vi "GetHighPrioritySensors.vi"() -> ()   [LabVIEW 2019]
uses:
  refnums.vi
  sensors.vi
  dsdata.vi
  <vilib>/Utility/xml.llb/Write to XML File(string).vi
  <vilib>/Utility/xml.llb/Read From XML File(array).vi
panel:
  in  "Plot":bool
  out "Drive Encoder Velocities":T1(graph)
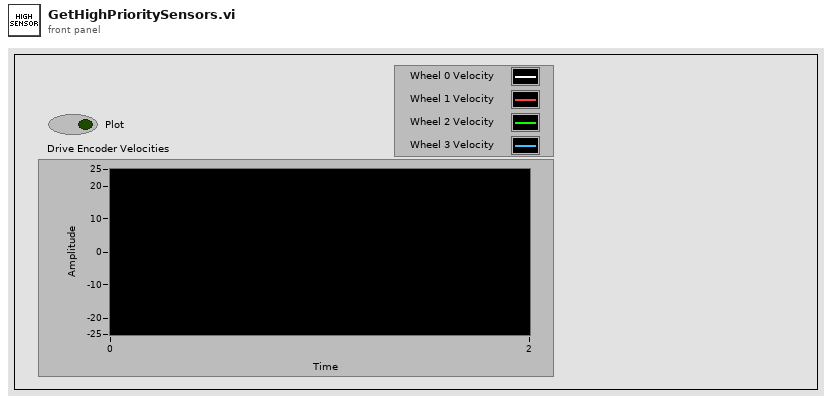
[diagram p1: front panel]
types:
  T1 = cluster{"Sensor Velocity":dbl, "Sensor Velocity":dbl, "Sensor Velocity":dbl, "Sensor Velocity":dbl}
  T2 = typedef "WPI_MotorControlDeviceRef.ctl" = cluster{"DeviceStatus":errorcluster, "Type":T3, "PWM":cluster{"PWM Channel":T4, "DeadBand":T5}, "CAN":cluster{"Device Number":u8, "SetOutput VI Ref":variant, "GetOutput VI Ref":variant, "Enable VI Ref":variant, "Disable VI Ref":variant, "Data":variant}, "Invert":bool, "DIO PWM":cluster{"PWM \"Enable\" Channel":T4, "DIOChannel":T6, "PWM Rate":dbl}}
  T3 = typedef "WPI_MotorControlType.ctl" = enum16{"PWM", "CAN", "DIO PWM"}
  T4 = typedef "FPGA_DIOPWMChannel.ctl" = enum8{"PWM 0", "PWM 1", "PWM 2", "PWM 3", "PWM 4", "PWM 5", "PWM 6", "PWM 7", "PWM 8", "PWM 9", "PWM MXP 0", "PWM MXP 1", "PWM MXP 2", "PWM MXP 3", "PWM MXP 4", "PWM MXP 5", "PWM MXP 6", "PWM MXP 7", "PWM MXP 8", "PWM MXP 9", "Invalid"}
  T5 = typedef "WPI_PWMDeadband.ctl" = cluster{"Name":string, "maxPositivePwm":i32, "minPositivePwm":i32, "centerPwm":i32, "maxNegativePwm":i32, "minNegativePwm":i32, "angularRange":u16}
  T6 = typedef "FPGA_DIOChannel.ctl" = enum8{"DIO 0", "DIO 1", "DIO 2", "DIO 3", "DIO 4", "DIO 5", "DIO 6", "DIO 7", "DIO 8", "DIO 9", "DIO MXP 0", "DIO MXP 1", "DIO MXP 2", "DIO MXP 3", "DIO MXP 4", "DIO MXP 5", "DIO MXP 6", "DIO MXP 7", "DIO MXP 8", "DIO MXP 9", "DIO MXP 10", "DIO MXP 11", "DIO MXP 12", "DIO MXP 13", "DIO MXP 14", "DIO MXP 15", "SPI Port CS1", "SPI Port CS2", "SPI Port CS3", "SPI Port MISO", "SPI Port MOSI", "Invalid"}
  T7 = typedef "WPI_PotentiometerDevRef.ctl" = cluster{"DevStatus":errorcluster, "Analog Channel":T8, "Invert Output":bool}
  T8 = typedef "FPGA_AIChannel.ctl" = enum8{"AI 0", "AI 1", "AI 2", "AI 3", "AI MXP 0", "AI MXP 1", "AI MXP 2", "AI MXP 3", "Invalid"}
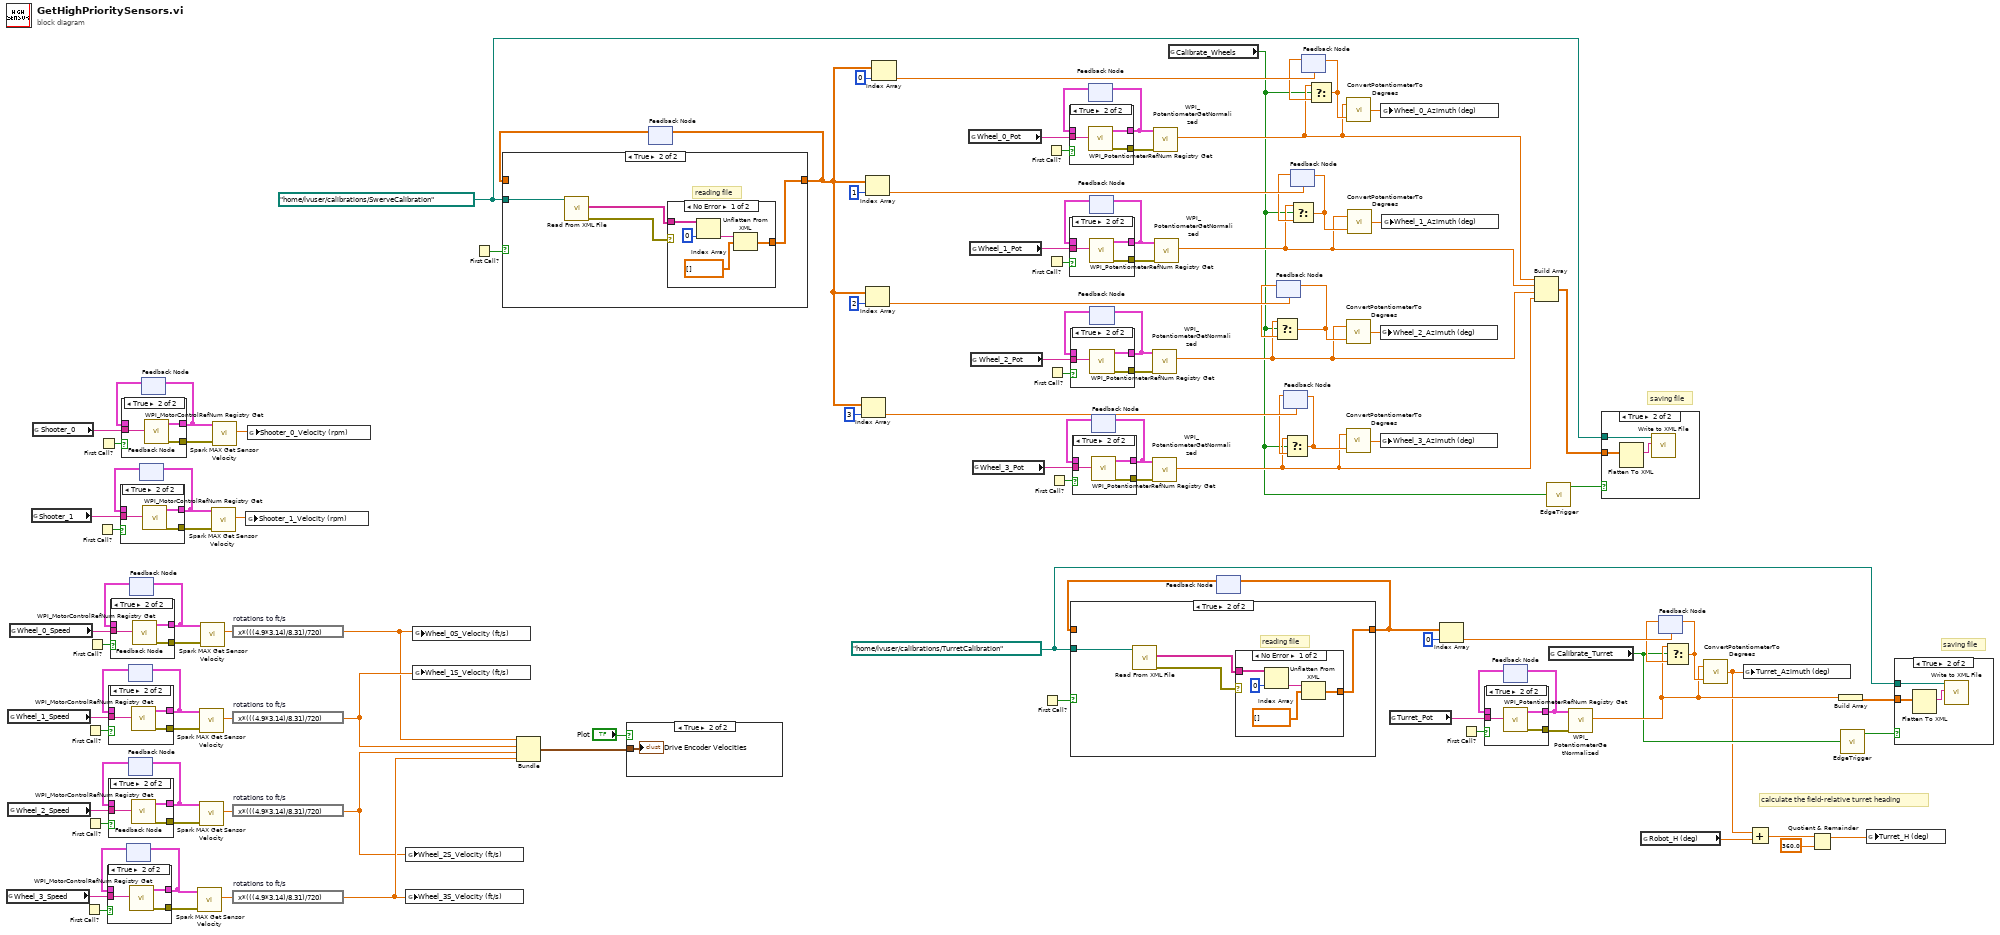
[diagram p0: block diagram]
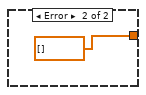
[diagram p4: hidden frame]
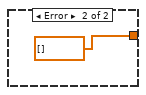
[diagram p15: hidden frame]
diagram:
  w8 = path "/home/lvuser/calibrations/TurretCalibration" ("path")
  w67 = path "/home/lvuser/calibrations/SwerveCalibration" ("path")
  # "calculate the field-relative turret heading"
  # "saving file"
  # "saving file"
  n1 = global read "refnums.vi" "Wheel_3_Speed"() -> (w33:string)
  n2 = global read "refnums.vi" "Wheel_1_Speed"() -> (w43:string)
  n3 = global read "refnums.vi" "Wheel_2_Speed"() -> (w38:string)
  n4 = global read "refnums.vi" "Wheel_0_Speed"() -> (w48:string)
  n5 = global read "refnums.vi" "Shooter_1"() -> (w56:string)
  n6 = global read "refnums.vi" "Shooter_0"() -> (w62:string)
  n7 = First Call?() -> (First Call?: T/F=w35:bool)
  n8 = First Call?() -> (First Call?: T/F=w45:bool)
  n9 = First Call?() -> (First Call?: T/F=w40:bool)
  n10 = First Call?() -> (First Call?: T/F=w50:bool)
  n11 = First Call?() -> (First Call?: T/F=w58:bool)
  n12 = First Call?() -> (First Call?: T/F=w64:bool)
  n13 = feedback #1() -> (w34:T2)  [unwired: 1 in]
  n14 = case shown="True" w35 {
    tunnel: [w116 w119] -> w31
    tunnel: w34 -> [w116 _]
    tunnel: w33 -> [_ w117]
    tunnel: [_ w118] -> w32
    frame False {
    }
    frame True {
      n15 = call <vilib>:"WPI_MotorControlRefNum Registry Get.vi"("refnum name"=w117) -> ("error out"=w118:errorcluster, "MotorControlDevRef"=w119:T2)  [unwired: 9 in]
    }
  }
  n16 = feedback-in #1(w31) -> ()
  n17 = feedback #2() -> (w44:T2)  [unwired: 1 in]
  n18 = case shown="True" w45 {
    tunnel: [w120 w123] -> w41
    tunnel: w44 -> [w120 _]
    tunnel: w43 -> [_ w121]
    tunnel: [_ w122] -> w42
    frame False {
    }
    frame True {
      n19 = call <vilib>:"WPI_MotorControlRefNum Registry Get.vi"("refnum name"=w121) -> ("error out"=w122:errorcluster, "MotorControlDevRef"=w123:T2)  [unwired: 9 in]
    }
  }
  n20 = feedback-in #2(w41) -> ()
  n21 = feedback #3() -> (w39:T2)  [unwired: 1 in]
  n22 = case shown="True" w40 {
    tunnel: [w124 w127] -> w36
    tunnel: w39 -> [w124 _]
    tunnel: w38 -> [_ w125]
    tunnel: [_ w126] -> w37
    frame False {
    }
    frame True {
      n23 = call <vilib>:"WPI_MotorControlRefNum Registry Get.vi"("refnum name"=w125) -> ("error out"=w126:errorcluster, "MotorControlDevRef"=w127:T2)  [unwired: 9 in]
    }
  }
  n24 = feedback-in #3(w36) -> ()
  n25 = feedback #4() -> (w49:T2)  [unwired: 1 in]
  n26 = case shown="True" w50 {
    tunnel: [w128 w131] -> w46
    tunnel: w49 -> [w128 _]
    tunnel: w48 -> [_ w129]
    tunnel: [_ w130] -> w47
    frame False {
    }
    frame True {
      n27 = call <vilib>:"WPI_MotorControlRefNum Registry Get.vi"("refnum name"=w129) -> ("error out"=w130:errorcluster, "MotorControlDevRef"=w131:T2)  [unwired: 9 in]
    }
  }
  n28 = feedback-in #4(w46) -> ()
  n29 = feedback #5() -> (w57:T2)  [unwired: 1 in]
  n30 = case shown="True" w58 {
    tunnel: [w132 w135] -> w54
    tunnel: w57 -> [w132 _]
    tunnel: w56 -> [_ w133]
    tunnel: [_ w134] -> w55
    frame False {
    }
    frame True {
      n31 = call <vilib>:"WPI_MotorControlRefNum Registry Get.vi"("refnum name"=w133) -> ("error out"=w134:errorcluster, "MotorControlDevRef"=w135:T2)  [unwired: 9 in]
    }
  }
  n32 = feedback-in #5(w54) -> ()
  n33 = feedback #6() -> (w63:T2)  [unwired: 1 in]
  n34 = case shown="True" w64 {
    tunnel: [w136 w139] -> w60
    tunnel: w63 -> [w136 _]
    tunnel: w62 -> [_ w137]
    tunnel: [_ w138] -> w61
    frame False {
    }
    frame True {
      n35 = call <vilib>:"WPI_MotorControlRefNum Registry Get.vi"("refnum name"=w137) -> ("error out"=w138:errorcluster, "MotorControlDevRef"=w139:T2)  [unwired: 9 in]
    }
  }
  n36 = feedback-in #6(w60) -> ()
  n37 = call <vilib>:"Spark MAX Get Sensor Velocity.vi"("error in (no error)"=w32, "MotorControlDevRef in"=w31) -> ("Sensor Velocity"=w30:dbl)  [unwired: 6 in, 3 out]
  n38 = call <vilib>:"Spark MAX Get Sensor Velocity.vi"("error in (no error)"=w42, "MotorControlDevRef in"=w41) -> ("Sensor Velocity"=w26:dbl)  [unwired: 6 in, 3 out]
  n39 = call <vilib>:"Spark MAX Get Sensor Velocity.vi"("error in (no error)"=w37, "MotorControlDevRef in"=w36) -> ("Sensor Velocity"=w28:dbl)  [unwired: 6 in, 3 out]
  n40 = call <vilib>:"Spark MAX Get Sensor Velocity.vi"("error in (no error)"=w47, "MotorControlDevRef in"=w46) -> ("Sensor Velocity"=w23:dbl)  [unwired: 6 in, 3 out]
  n41 = call <vilib>:"Spark MAX Get Sensor Velocity.vi"("error in (no error)"=w55, "MotorControlDevRef in"=w54) -> ("Sensor Velocity"=w53:dbl)  [unwired: 6 in, 3 out]
  n42 = call <vilib>:"Spark MAX Get Sensor Velocity.vi"("error in (no error)"=w61, "MotorControlDevRef in"=w60) -> ("Sensor Velocity"=w59:dbl)  [unwired: 6 in, 3 out]
  n43 = expression code="x*(((4.9*3.14)/8.31)/720)" "rotations to ft/s"(w23) -> (w24:dbl)
  n44 = expression code="x*(((4.9*3.14)/8.31)/720)" "rotations to ft/s"(w26) -> (w25:dbl)
  n45 = expression code="x*(((4.9*3.14)/8.31)/720)" "rotations to ft/s"(w28) -> (w27:dbl)
  n46 = expression code="x*(((4.9*3.14)/8.31)/720)" "rotations to ft/s"(w30) -> (w29:dbl)
  n47 = global write "sensors.vi" "Shooter_1_Velocity (rpm)"(w53) -> ()
  n48 = global write "sensors.vi" "Shooter_0_Velocity (rpm)"(w59) -> ()
  n49 = global write "sensors.vi" "Wheel_2S_Velocity (ft/s)"(w27) -> ()
  n50 = global write "sensors.vi" "Wheel_3S_Velocity (ft/s)"(w29) -> ()
  n51 = global write "sensors.vi" "Wheel_0S_Velocity (ft/s)"(w24) -> ()
  n52 = global write "sensors.vi" "Wheel_1S_Velocity (ft/s)"(w25) -> ()
  n53 = First Call?() -> (First Call?: T/F=w73:bool)
  n54 = Bundle("Sensor Velocity"=w24, "Sensor Velocity"=w25, "Sensor Velocity"=w27, "Sensor Velocity"=w29) -> (w52:T1)  [unwired: 1 in]
  n55 = case shown="True" "Plot" {
    tunnel: w52 -> [_ w140]
    frame False {
    }
    frame True {
      "Drive Encoder Velocities" <- w140
    }
  }
  n56 = feedback #7() -> (w88:dbl[])  [unwired: 1 in]
  n57 = case shown="True" w73 {
    tunnel: w67 -> [_ w145]
    tunnel: [w141 w142] -> w79
    tunnel: w88 -> [w141 _]
    frame False {
    }
    frame True {
      # "reading file"
      n58 = call-poly <vilib>:"Read From XML File.vi"("XML File Path"=w145) -> ("error out"=w143:errorcluster, "XML Elements"=w144:string[])  [unwired: 8 in, 1 out]
      n59 = case shown="No Error" w143 {
        tunnel: w144 -> [w149 _]
        tunnel: [w147 dbl[] [] ("appended array")] -> w142
        frame No Error {
          n60 = Index Array(array=w149, index=0) -> (element=w148:string)
          n61 = Unflatten From XML(xml string=w148, type=dbl[] [] ("appended array")) -> (value=w147:dbl[])  [unwired: 1 in, 1 out]
        }
        frame Error {
        }
      }
    }
  }
  n62 = feedback-in #7(w79) -> ()
  n63 = Index Array(array=w79, index=3) -> (element=w81:dbl)
  n64 = Index Array(array=w79, index=1) -> (element=w86:dbl)
  n65 = Index Array(array=w79, index=2) -> (element=w83:dbl)
  n66 = Index Array(array=w79, index=0) -> (element=w90:dbl)
  n67 = global read "refnums.vi" "Wheel_0_Pot"() -> (w109:string)
  n68 = global read "refnums.vi" "Wheel_1_Pot"() -> (w105:string)
  n69 = global read "refnums.vi" "Wheel_2_Pot"() -> (w99:string)
  n70 = global read "refnums.vi" "Wheel_3_Pot"() -> (w94:string)
  n71 = First Call?() -> (First Call?: T/F=w11:bool)
  n72 = First Call?() -> (First Call?: T/F=w111:bool)
  n73 = First Call?() -> (First Call?: T/F=w107:bool)
  n74 = First Call?() -> (First Call?: T/F=w101:bool)
  n75 = First Call?() -> (First Call?: T/F=w96:bool)
  n76 = feedback #8() -> (w110:T7)  [unwired: 1 in]
  n77 = case shown="True" w111 {
    tunnel: [w152 w154] -> w108
    tunnel: w110 -> [w152 _]
    tunnel: w109 -> [_ w155]
    tunnel: [_ w153] -> w104
    frame False {
    }
    frame True {
      n78 = call <vilib>:"WPI_PotentiometerRefNum Registry Get.vi"("refnum name"=w155) -> ("error out"=w153:errorcluster, "PotDevRef"=w154:T7)  [unwired: 9 in]
    }
  }
  n79 = feedback-in #8(w108) -> ()
  n80 = feedback #9() -> (w106:T7)  [unwired: 1 in]
  n81 = case shown="True" w107 {
    tunnel: [w156 w158] -> w103
    tunnel: w106 -> [w156 _]
    tunnel: w105 -> [_ w159]
    tunnel: [_ w157] -> w102
    frame False {
    }
    frame True {
      n82 = call <vilib>:"WPI_PotentiometerRefNum Registry Get.vi"("refnum name"=w159) -> ("error out"=w157:errorcluster, "PotDevRef"=w158:T7)  [unwired: 9 in]
    }
  }
  n83 = feedback-in #9(w103) -> ()
  n84 = feedback #10() -> (w100:T7)  [unwired: 1 in]
  n85 = case shown="True" w101 {
    tunnel: [w160 w162] -> w98
    tunnel: w100 -> [w160 _]
    tunnel: w99 -> [_ w163]
    tunnel: [_ w161] -> w97
    frame False {
    }
    frame True {
      n86 = call <vilib>:"WPI_PotentiometerRefNum Registry Get.vi"("refnum name"=w163) -> ("error out"=w161:errorcluster, "PotDevRef"=w162:T7)  [unwired: 9 in]
    }
  }
  n87 = feedback-in #10(w98) -> ()
  n88 = feedback #11() -> (w95:T7)  [unwired: 1 in]
  n89 = case shown="True" w96 {
    tunnel: [w164 w166] -> w93
    tunnel: w95 -> [w164 _]
    tunnel: w94 -> [_ w167]
    tunnel: [_ w165] -> w92
    frame False {
    }
    frame True {
      n90 = call <vilib>:"WPI_PotentiometerRefNum Registry Get.vi"("refnum name"=w167) -> ("error out"=w165:errorcluster, "PotDevRef"=w166:T7)  [unwired: 9 in]
    }
  }
  n91 = feedback-in #11(w93) -> ()
  n92 = call <vilib>:"WPI_PotentiometerGetNormalized.vi"("error in"=w97, "PotDevRef"=w98) -> ("Normalized Value"=w70:dbl)  [unwired: 7 in, 2 out]
  n93 = call <vilib>:"WPI_PotentiometerGetNormalized.vi"("error in"=w92, "PotDevRef"=w93) -> ("Normalized Value"=w69:dbl)  [unwired: 7 in, 2 out]
  n94 = call <vilib>:"WPI_PotentiometerGetNormalized.vi"("error in"=w104, "PotDevRef"=w108) -> ("Normalized Value"=w68:dbl)  [unwired: 7 in, 2 out]
  n95 = call <vilib>:"WPI_PotentiometerGetNormalized.vi"("error in"=w102, "PotDevRef"=w103) -> ("Normalized Value"=w71:dbl)  [unwired: 7 in, 2 out]
  n96 = global read "dsdata.vi" "Calibrate_Wheels"() -> (w66:bool)
  n97 = feedback #12() -> (w14:dbl[])  [unwired: 1 in]
  n98 = case shown="True" w11 {
    tunnel: w8 -> [_ w172]
    tunnel: [w168 w169] -> w13
    tunnel: w14 -> [w168 _]
    frame False {
    }
    frame True {
      # "reading file"
      n99 = call-poly <vilib>:"Read From XML File.vi"("XML File Path"=w172) -> ("error out"=w170:errorcluster, "XML Elements"=w171:string[])  [unwired: 8 in, 1 out]
      n100 = case shown="No Error" w170 {
        tunnel: w171 -> [w176 _]
        tunnel: [w174 dbl[] [] ("appended array")] -> w169
        frame No Error {
          n101 = Index Array(array=w176, index=0) -> (element=w175:string)
          n102 = Unflatten From XML(xml string=w175, type=dbl[] [] ("appended array")) -> (value=w174:dbl[])  [unwired: 1 in, 1 out]
        }
        frame Error {
        }
      }
    }
  }
  n103 = feedback-in #12(w13) -> ()
  n104 = feedback #13(w83) -> (w82:dbl)
  n105 = Select(t=w70, s=w66, f=w82) -> (s? t:f=w75:dbl)
  n106 = feedback-in #13(w75) -> ()
  n107 = feedback #14(w81) -> (w80:dbl)
  n108 = Select(t=w69, s=w66, f=w80) -> (s? t:f=w74:dbl)
  n109 = feedback-in #14(w74) -> ()
  n110 = feedback #15(w86) -> (w85:dbl)
  n111 = Select(t=w71, s=w66, f=w85) -> (s? t:f=w76:dbl)
  n112 = feedback-in #15(w76) -> ()
  n113 = feedback #16(w90) -> (w89:dbl)
  n114 = Select(t=w68, s=w66, f=w89) -> (s? t:f=w77:dbl)
  n115 = feedback-in #16(w77) -> ()
  n116 = call "ConvertPotentiometerToDegrees.vi"("Forward Position Wheel 1 [0-1]"=w75, "Raw Potentiometer Value"=w70) -> ("Orientation (deg)"=w113:dbl)
  n117 = call "ConvertPotentiometerToDegrees.vi"("Forward Position Wheel 1 [0-1]"=w74, "Raw Potentiometer Value"=w69) -> ("Orientation (deg)"=w112:dbl)
  n118 = call "ConvertPotentiometerToDegrees.vi"("Forward Position Wheel 1 [0-1]"=w77, "Raw Potentiometer Value"=w68) -> ("Orientation (deg)"=w115:dbl)
  n119 = call "ConvertPotentiometerToDegrees.vi"("Forward Position Wheel 1 [0-1]"=w76, "Raw Potentiometer Value"=w71) -> ("Orientation (deg)"=w114:dbl)
  n120 = global write "sensors.vi" "Wheel_2_Azimuth (deg)"(w113) -> ()
  n121 = global write "sensors.vi" "Wheel_3_Azimuth (deg)"(w112) -> ()
  n122 = global write "sensors.vi" "Wheel_0_Azimuth (deg)"(w115) -> ()
  n123 = global write "sensors.vi" "Wheel_1_Azimuth (deg)"(w114) -> ()
  n124 = global read "refnums.vi" "Turret_Pot"() -> (w20:string)
  n125 = Index Array(array=w13, index=0) -> (element=w16:dbl)
  n126 = First Call?() -> (First Call?: T/F=w22:bool)
  n127 = feedback #17() -> (w21:T7)  [unwired: 1 in]
  n128 = case shown="True" w22 {
    tunnel: [w179 w181] -> w19
    tunnel: w21 -> [w179 _]
    tunnel: w20 -> [_ w182]
    tunnel: [_ w180] -> w18
    frame False {
    }
    frame True {
      n129 = call <vilib>:"WPI_PotentiometerRefNum Registry Get.vi"("refnum name"=w182) -> ("error out"=w180:errorcluster, "PotDevRef"=w181:T7)  [unwired: 9 in]
    }
  }
  n130 = feedback-in #17(w19) -> ()
  n131 = Build Array(w68, w71, w70, w69) -> (w72:dbl[])
  n132 = call "EdgeTrigger.vi"("Input Signal"=w66) -> ("Rising Edge Trigger"=w65:bool)  [unwired: 2 out]
  n133 = global read "dsdata.vi" "Calibrate_Turret"() -> (w6:bool)
  n134 = call <vilib>:"WPI_PotentiometerGetNormalized.vi"("error in"=w18, "PotDevRef"=w19) -> ("Normalized Value"=w9:dbl)  [unwired: 7 in, 2 out]
  n135 = case shown="True" w65 {
    tunnel: w67 -> [_ w185]
    tunnel: w72 -> [_ w184]
    frame False {
    }
    frame True {
      n136 = Flatten To XML(anything=w184) -> (xml string=w183:string)
      n137 = call-poly <vilib>:"Write to XML File.vi"("XML Input"=w183, "XML File Path"=w185) -> ()  [unwired: 7 in, 3 out]
    }
  }
  n138 = global read "sensors.vi" "Robot_H (deg)"() -> (w2:dbl)
  n139 = feedback #18(w16) -> (w15:dbl)
  n140 = Select(t=w9, s=w6, f=w15) -> (s? t:f=w12:dbl)
  n141 = feedback-in #18(w12) -> ()
  n142 = call "ConvertPotentiometerToDegrees.vi"("Forward Position Wheel 1 [0-1]"=w12, "Raw Potentiometer Value"=w9) -> ("Orientation (deg)"=w3:dbl)
  n143 = global write "sensors.vi" "Turret_Azimuth (deg)"(w3) -> ()
  n144 = Add(x=w3, y=w2) -> (x+y=w5:dbl)
  n145 = Quotient & Remainder(x=w5, y=360.0) -> (x-y*floor(x/y)=w1:dbl)  [unwired: 1 out]
  n146 = Build Array(w9) -> (w10:dbl[])
  n147 = call "EdgeTrigger.vi"("Input Signal"=w6) -> ("Rising Edge Trigger"=w7:bool)  [unwired: 2 out]
  n148 = global write "sensors.vi" "Turret_H (deg)"(w1) -> ()
  n149 = case shown="True" w7 {
    tunnel: w8 -> [_ w188]
    tunnel: w10 -> [_ w187]
    frame False {
    }
    frame True {
      n150 = Flatten To XML(anything=w187) -> (xml string=w186:string)
      n151 = call-poly <vilib>:"Write to XML File.vi"("XML Input"=w186, "XML File Path"=w188) -> ()  [unwired: 7 in, 3 out]
    }
  }
